vi "FV-resample-get_max_array_value.vi"(7 "max Frequency":dbl, 10 "Frequency array":dbl[](array[numeric])) -> (1 "Position":i32, 2 "cut array":dbl[](array[numeric]))   [LabVIEW 2020, in "FV-file_viewer.lvlib"]
uses:
  FV-file_viewer.lvlib
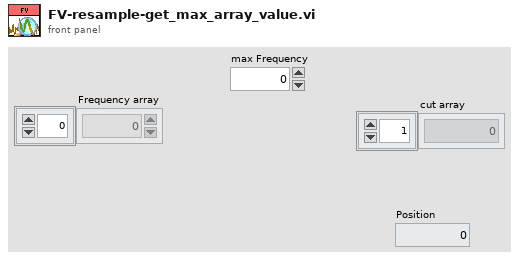
[diagram p1: front panel]
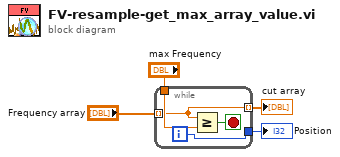
[diagram p0: block diagram]
diagram:
  n1 = while {
    tunnel: "Frequency array" -> [w6] mode=indexing
    tunnel: "max Frequency" -> [w8]
    tunnel: [w6] -> w1 mode=indexing
    tunnel: [w5] -> w2
    i -> [w5]
    stop <- w7 stop-if-true
    n2 = Greater Or Equal?(x=w6, y=w8) -> (x >= y?=w7:bool)
  }
  "Position" <- w2
  "cut array" <- w1
